vi "Write Datafile Path.vi"(8 "error in (no error)":errorcluster, 10 "Datafile Path":path, 11 "Controller in":refnum<class "Controller.lvclass">) -> (0 "error out":errorcluster, 3 "Controller out":refnum<class "Controller.lvclass">)   [LabVIEW 2019, in "Controller.lvlib" / "Controller.lvclass"]
uses:
  Controller.lvclass
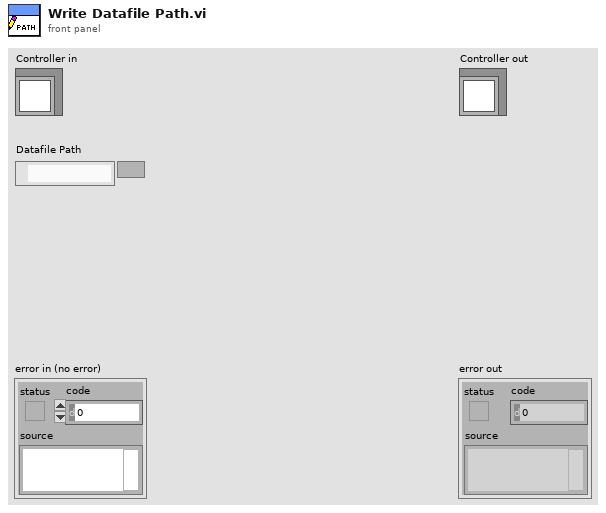
[diagram p1: front panel]
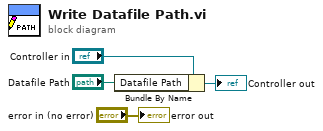
[diagram p0: block diagram]
diagram:
  n1 = Bundle By Name(cluster="Controller in", "Datafile Path"="Datafile Path") -> (→"Controller out":refnum<class "Controller.lvclass">)
  "error out" <- "error in (no error)"
